vi "ListSelectedSigArry.vi"(6 "SelectedSigValListArry":refnum<vi>, 7 "已选信号选择器":refnum<vi>, 8 "SigValListArry":refnum<vi>, 9 "全部信号数组":refnum<vi>, 10 "已选信号数组":refnum<vi>, 11 "已选列表":refnum<vi>) -> (1 "NoMpor":bool)   [LabVIEW 2015]
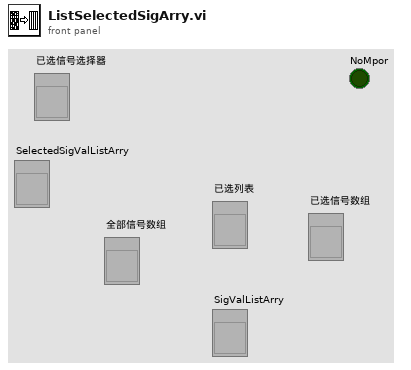
[diagram p1: front panel]
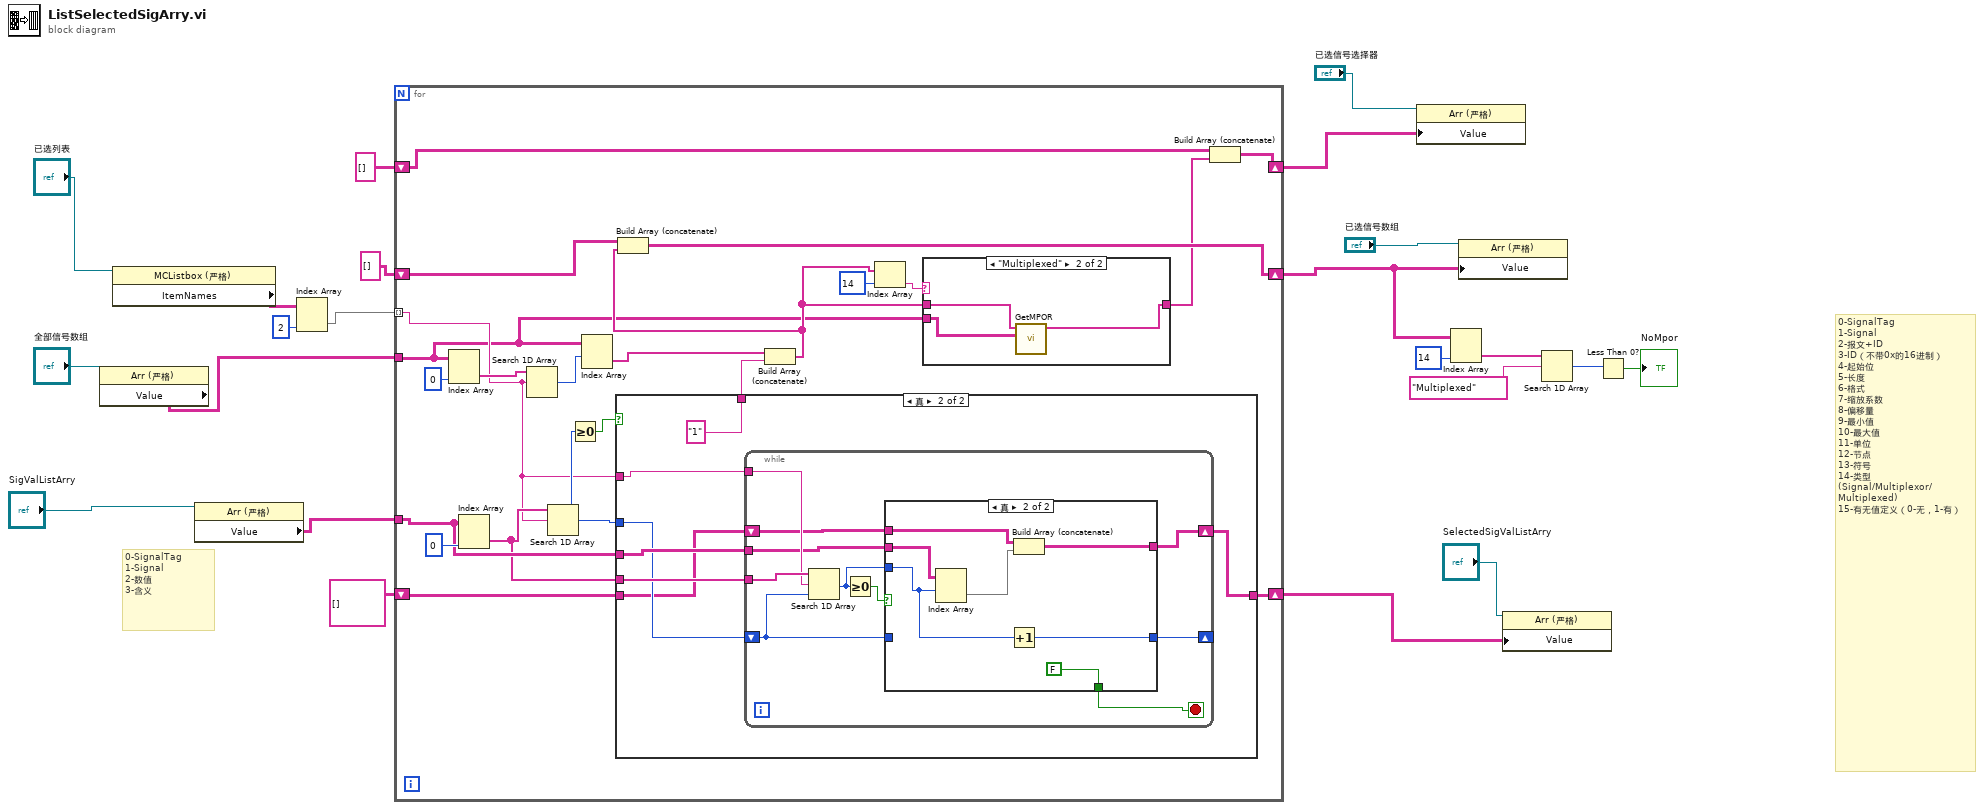
[diagram p0: block diagram]
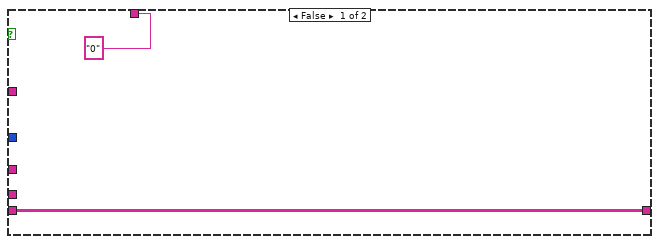
[diagram p3: hidden frame]
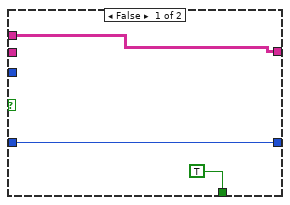
[diagram p4: hidden frame]
diagram:
  # "0-SignalTag\n1-Signal\n2-报文+ID\n3-ID（不带0x的16进制）\n4-起始位\n5-长度\n6-格式\n7-缩放系数\n8-偏移量\n9-最小值\n10-最大值\n11-单位\n12-节点\n13-符号\n14-类型\n(Signal/Multiplexor/\nMultiplexed)\n15-有无值定义（0-无，1-有）"
  # "0-SignalTag\n1-Signal\n2-数值\n3-含义"
  n1 = property class="Arr (严格)"(reference="全部信号数组") -> ("Value"=w22:string[][])  [unwired: 1 in, 2 out]
  n2 = property on="属性节点" class="MCListbox (严格)"(reference="已选列表") -> ("ItemNames"=w16:string[][])  [unwired: 1 in, 2 out]
  n3 = property class="Arr (严格)"(reference="SigValListArry") -> ("Value"=w13:string[][])  [unwired: 1 in, 2 out]
  n4 = Index Array(array=w16, index (col)=2 ("禁用的索引 (列)")) -> (element=w18:string[])  [unwired: 1 in]
  n5 = for {
    tunnel: w18 -> [w32] mode=indexing
    tunnel: w22 -> [w23]
    shift-right: [w41] -> w6
    shift-left: string[][] [] -> [w40]
    tunnel: w13 -> [w35]
    shift-right: [w30] -> w10
    shift-left: string[][] [] -> [w31]
    shift-right: [w28] -> w8
    shift-left: string[][] [] -> [w29]
    n6 = Index Array(array=w23, index (col)=0 ("禁用的索引 (列)")) -> (element=w43:string[])  [unwired: 1 in]
    n7 = Index Array(array=w35, index (col)=0 ("禁用的索引 (列)")) -> (element=w33:string[])  [unwired: 1 in]
    n8 = Search 1D Array(1D array=w43, element=w32) -> (index of element=w42:i32)  [unwired: 1 in]
    n9 = Search 1D Array(1D array=w33, element=w32) -> (index of element=w34:i32)  [unwired: 1 in]
    n10 = Greater Or Equal To 0?(x=w34) -> (x >= 0?=w38:bool)
    n11 = Index Array(array=w23, index (row)=w42) -> (element=w37:string[])  [unwired: 1 in]
    n12 = case shown="真" w38 {
      tunnel: ["0" "1"] -> w36
      tunnel: w35 -> [_ w54]
      tunnel: w34 -> [_ w53]
      tunnel: w33 -> [_ w56]
      tunnel: w32 -> [_ w55]
      tunnel: [w49 w52] -> w30
      tunnel: w31 -> [w49 w51]
      frame False {
      }
      frame True {
        n13 = while {
          tunnel: w56 -> [w67]
          tunnel: w55 -> [w66]
          tunnel: w54 -> [w64]
          shift-right: [w62] -> w52
          shift-left: w51 -> [w61]
          shift-right: [w60] -> _
          shift-left: w53 -> [w59]
          stop <- w58 stop-if-true
          n14 = Search 1D Array(1D array=w67, element=w66, start index (0)=w59) -> (index of element=w63:i32)
          n15 = Greater Or Equal To 0?(x=w63) -> (x >= 0?=w65:bool)
          n16 = case shown="真" w65 {
            tunnel: w64 -> [_ w77]
            tunnel: w63 -> [_ w73]
            tunnel: [w70 w75] -> w62
            tunnel: w61 -> [w70 w74]
            tunnel: [w69 w72] -> w60
            tunnel: w59 -> [w69 _]
            tunnel: [TRUE FALSE] -> w58
            frame False {
            }
            frame True {
              n17 = Index Array(array=w77, index (row)=w73) -> (element=w76:string[])  [unwired: 1 in]
              n18 = Increment(x=w73) -> (x+1=w72:i32)
              n19 = Build Array (concatenate)(w74, w76) -> (w75:string[][])
            }
          }
        }
      }
    }
    n20 = Build Array (concatenate)(w37, w36) -> (w25:string[])
    n21 = Build Array (concatenate)(w40, w25) -> (w41:string[][])
    n22 = Index Array(array=w25, index=14 ("索引")) -> (element=w26:string)
    n23 = case shown="\"Multiplexed\"" w26 {
      tunnel: w25 -> [w45 w46]
      tunnel: [w45 w47] -> w24
      tunnel: w23 -> [_ w48]
      frame "假", Default {
      }
      frame "Multiplexed" {
        n24 = call "GetMPOR.vi"("全部信号数组"=w48, "当前信号"=w46) -> ("MPOR"=w47:string[])  [unwired: 9 in]
      }
    }
    n25 = Build Array (concatenate)(w29, w24) -> (w28:string[][])
  }
  n26 = property class="Arr (严格)"(reference="已选信号选择器", "Value"=w8) -> ()  [unwired: 1 in, 2 out]
  n27 = Index Array(array=w6, index (col)=14 ("禁用的索引 (列)")) -> (element=w4:string[])  [unwired: 1 in]
  n28 = property class="Arr (严格)"(reference="已选信号数组", "Value"=w6) -> ()  [unwired: 1 in, 2 out]
  n29 = property class="Arr (严格)"(reference="SelectedSigValListArry", "Value"=w10) -> ()  [unwired: 1 in, 2 out]
  n30 = Search 1D Array(1D array=w4, element="Multiplexed" ("元素")) -> (index of element=w2:i32)  [unwired: 1 in]
  n31 = Less Than 0?(x=w2) -> (x < 0?=→"NoMpor":bool)
